vi "spi_single_master.vi"(7 "Falling Edge?":bool=TRUE, 8 "SIG Port":refnum<k21>="Connector0/DIO0", 9 "CLK Port":refnum<k21>="Connector0/DIO1", 11 "Signal":bool=TRUE) -> (0 "SIG Port Out":refnum<k21>="Connector0/DIO0", 1 "CLK Port Out":refnum<k21>="Connector0/DIO1")   [LabVIEW 2016, in "kevLib2010.lvlib"]
uses:
  kevLib2010.lvlib
  <vilib>/rvi/eio/common/nirviEmuTemplateMethod_errors.vi
  <vilib>/eio/EIONode/EIONode.xnode
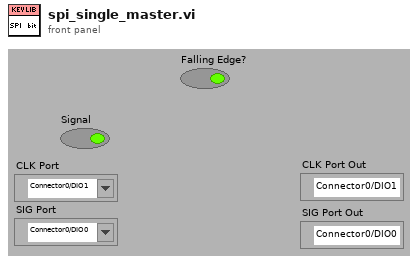
[diagram p1: front panel]
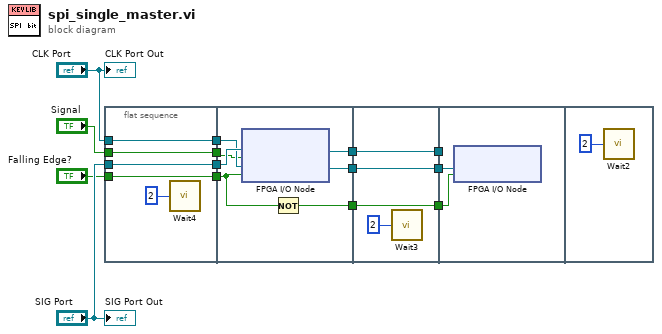
[diagram p0: block diagram]
diagram:
  n1 = flat-sequence {
    tunnel: "Signal" -> [w16]
    tunnel: "Falling Edge?" -> [w17]
    tunnel: "CLK Port" -> [w18]
    tunnel: "SIG Port" -> [w19]
    tunnel: [w19] -> w4
    tunnel: [w18] -> w3
    tunnel: [w17] -> w2
    tunnel: [w16] -> w1
    tunnel: [w24] -> w10
    tunnel: [w23] -> w8
    tunnel: [w21] -> w6
    tunnel: w4 -> [w26]
    tunnel: w3 -> [w25]
    tunnel: w2 -> [w22]
    tunnel: w1 -> [w20]
    tunnel: w10 -> [w30]
    tunnel: [w30] -> w9
    tunnel: w8 -> [w29]
    tunnel: [w29] -> w7
    tunnel: w6 -> [w28]
    tunnel: [w28] -> w5
    tunnel: w9 -> [_]
    tunnel: w7 -> [w32]
    tunnel: w5 -> [w31]
    frame #0 {
      n2 = call "Wait4"("Count(Ticks)"=u8 2) -> ()  [unwired: 1 out]
    }
    frame #1 {
      n3 = xnode "FPGA I/O Node"("I/O Item"=w20, "FPGA I/O In"=w26, "I/O Item"=w22, "FPGA I/O In"=w25) -> ("FPGA I/O Out"=w24:refnum<k21>, "FPGA I/O Out"=w23:refnum<k21>)
      n4 = Not(x=w22) -> (.not. x?=w21:bool)
    }
    frame #2 {
      n5 = call "Wait3"("Count(Ticks)"=u8 2) -> ()  [unwired: 1 out]
    }
    frame #3 {
      n6 = xnode "FPGA I/O Node"("I/O Item"=w31, "FPGA I/O In"=w32) -> ()  [unwired: 1 out]
    }
    frame #4 {
      n7 = call "Wait2"("Count(Ticks)"=u8 2) -> ()  [unwired: 1 out]
    }
  }
  "SIG Port Out" <- "SIG Port"
  "CLK Port Out" <- "CLK Port"
